vi "SpeedControlMotor4.vi"() -> ()   [LabVIEW 2014]
doc: "This example demonstrates how to simulate a general PID controller with a plant with noise."
uses:
  MyRIO Software/MyTypeDefs/EncoderController.ctl
  <vilib>/Analysis/3filter.llb/Filter Passband Type.ctl
  <vilib>/addons/control/pid/pid.llb/PID Percentage to EGU (DBL).vi
  <vilib>/addons/control/pid/pid.llb/PID Control Input Filter (DBL).vi
  <vilib>/addons/control/pid/pid.llb/PID (DBL).vi
  <vilib>/addons/control/pid/pid.llb/PID Output Rate Limiter (DBL).vi
  <vilib>/addons/control/pid/NI_PID_pid.lvlib
  <vilib>/ptbypt/NI_PtbyPt.lvlib
  <vilib>/Analysis/NI_AALBase.lvlib
panel:
  in  "Encoder 4 Controller":T1={"Sample time (uS)"=100000, "Reset"=FALSE}
  out "Sampling frequency (Hz)":dbl=4.0
  in  "cut-off frequency":dbl=6.0
  in  "order":i32=5
  in  "Filtering option":T2(ring)
  out "Manipulated variable (MV)":dbl(graph)=44.75756470842677
  in  "Output Limiter":bool
  in  "Output Rate (EGU/min)":dbl=10000.0 format="%#.2f"
  out "Unfiltered Speed(RPM)":dbl=55.83860880961906 format="%.4f"
  in  "Setpoint (RPM)":dbl(slide)=55.55555555555556 min=0.0 max=0.0 scale=-100.0..100.0
  out "MV:":dbl(slide)=38.025391430574594 scale=-100.0..100.0
  out "Speed (RPM):":dbl(slide)=55.83860880961906 scale=-100.0..100.0
  in  "PID gains":T3={"proportional gain (Kc)"=0.6, "integral time (Ti, min)"=0.01, "derivative time (Td, min)"=0.0} {"derivative time (Td, min)" format="%.3f"; "integral time (Ti, min)" format="%.3f"; "proportional gain (Kc)" format="%.3f"}
  in  "Controller Sampling Time":dbl=0.25 min=0.001 step=0.01 format="%#.3p"
  in  "Stop":bool
  out "System Monitor":T4(graph)={"Speed (RPM):"=55.13720442402905, "Setpoint (RPM)"=55.55555555555556, "Velocity RPM"=55.83860880961906}
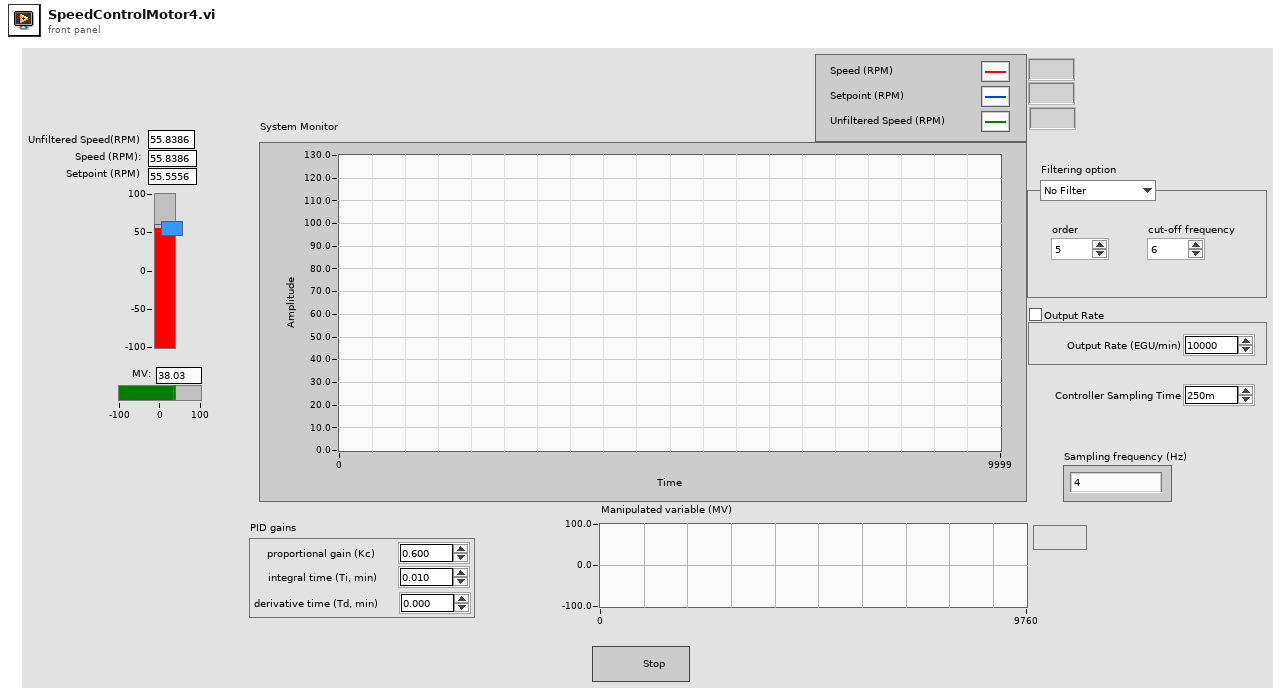
[diagram p1: front panel]
types:
  T1 = typedef "EncoderController.ctl" = cluster{"Sample time (uS)":u32, "Reset":bool}
  T2 = enum16{"No Filter", "PID FIR Filter", "Butterworth", "Chebyshev", "FIR Windowing", "Median"}
  T3 = cluster{"proportional gain (Kc)":dbl, "integral time (Ti, min)":dbl, "derivative time (Td, min)":dbl}
  T4 = cluster{"Speed (RPM):":dbl, "Setpoint (RPM)":dbl, "Velocity RPM":dbl}
  T5 = typedef "NI_AALBase.lvlib/Filter Passband Type.ctl" = enum32{"Lowpass", "Highpass", "Bandpass", "Bandstop"}
  T6 = cluster{bool, "Tick Count(uSec)":u32, "Counter Value":i32, "x-y":i32}
  T7 = typedef "EncoderIndicator.ctl" = cluster{"Position":dbl, "Velocity RPM":dbl, "Velocity RPS":dbl}
  T8 = cluster{"Speed (RPM):":dbl, "Setpoint (RPM)":dbl, dbl}
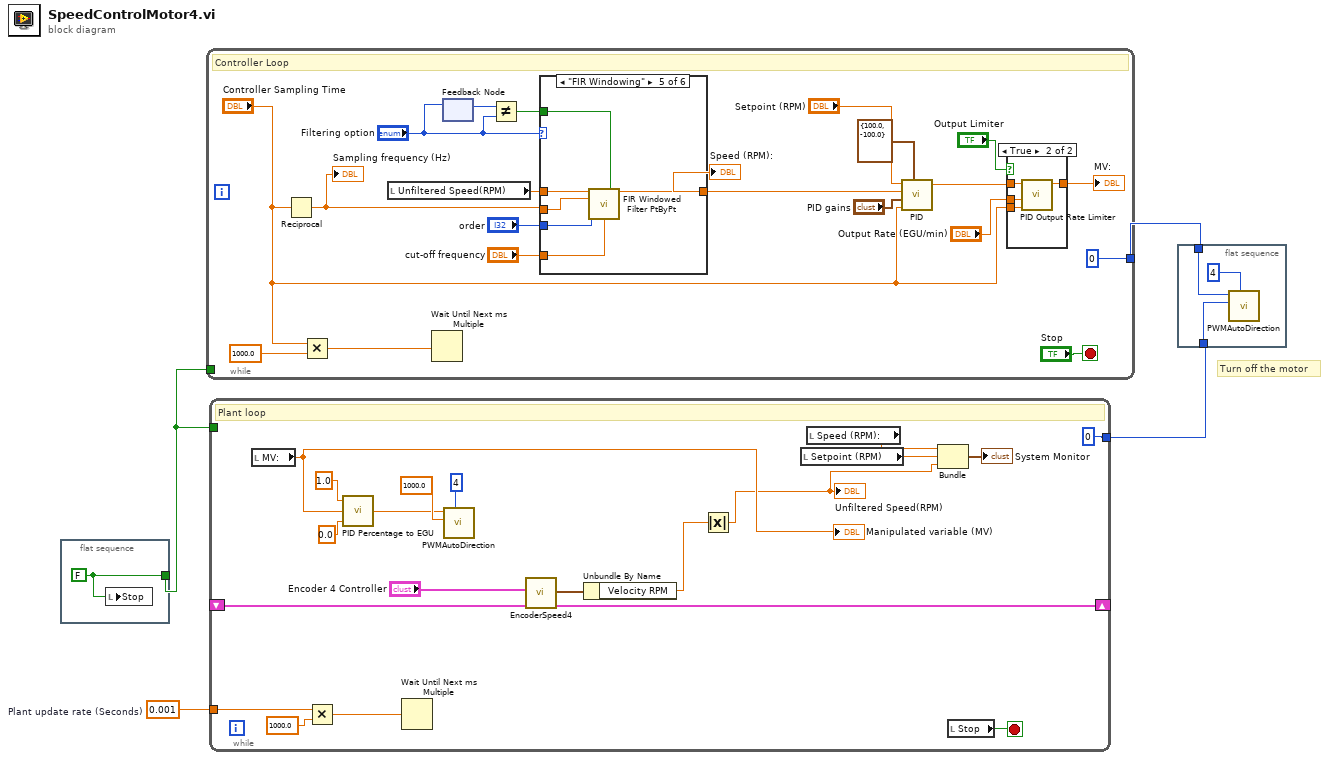
[diagram p0: block diagram]
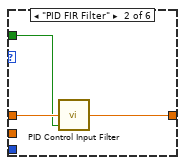
[diagram p3: hidden frame]
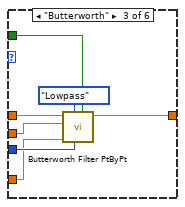
[diagram p4: hidden frame]
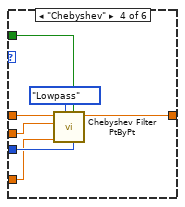
[diagram p5: hidden frame]
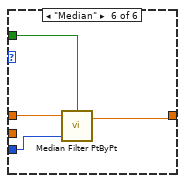
[diagram p6: hidden frame]
diagram:
  w4 = 0.001  # Plant update rate (Seconds)
  # "Turn off the motor"
  n1 = flat-sequence {
    tunnel: [w5] -> w3
    frame #0 {
      w5 = FALSE ("STOP")
      n2 = local write "Stop"(w5) -> ()
    }
  }
  n3 = while {
    tunnel: w3 -> [_]
    tunnel: [0] -> w2
    stop <- "Stop" stop-if-true
    # "Controller Loop"
    n4 = Reciprocal(x="Controller Sampling Time") -> (1/x=w24:dbl)
    "Sampling frequency (Hz)" <- w24
    n5 = Multiply(x="Controller Sampling Time", y=1000.0) -> (x*y=w25:dbl)
    n6 = local read "Unfiltered Speed(RPM)"() -> (w20:dbl)
    n7 = Wait Until Next ms Multiple(millisecond multiple=w25) -> ()  [unwired: 1 out]
    n8 = feedback-in #1("Filtering option") -> ()
    n9 = feedback #1() -> (w14:T2)  [unwired: 1 in]
    n10 = Not Equal?(x=w14, y="Filtering option") -> (x != y?=w12:bool)
    n11 = case shown="\"FIR Windowing\"" "Filtering option" {
      tunnel: [w26 w29 w36 w43 w49 w53] -> w21
      tunnel: w20 -> [w26 w28 w35 w42 w48 w52]
      tunnel: w24 -> [_ _ w34 w41 w47 _]
      tunnel: "order" -> [_ _ w32 w39 w46 w51]
      tunnel: "cut-off frequency" -> [_ _ w31 w38 w45 _]
      tunnel: w12 -> [_ w27 w30 w37 w44 w50]
      frame "No Filter", Default {
      }
      frame "PID FIR Filter" {
        n12 = call-poly <vilib>:"PID Control Input Filter.vi"("reinitialize? (F)"=w27, "input"=w28) -> ("output"=w29:dbl)  [unwired: 3 in]
      }
      frame "Butterworth" {
        n13 = call <vilib>:"Butterworth Filter PtByPt.vi"("initialize"=w30, "order"=w32, "filter type"=Filter_Passband_Type."Lowpass", "low cutoff freq: fl"=w31, "sampling freq: fs"=w34, "x"=w35) -> ("Filtered x"=w36:dbl)  [unwired: 3 in, 1 out]
      }
      frame "Chebyshev" {
        n14 = call <vilib>:"Chebyshev Filter PtByPt.vi"("order"=w39, "initialize"=w37, "filter type"=Filter_Passband_Type."Lowpass", "low cutoff freq: fl"=w38, "sampling freq: fs"=w41, "x"=w42) -> ("Filtered x"=w43:dbl)  [unwired: 4 in, 1 out]
      }
      frame "FIR Windowing" {
        n15 = call <vilib>:"FIR Windowed Filter PtByPt.vi"("x"=w48, "initialize"=w44, "sampling freq: fs"=w47, "taps"=w46, "low cutoff freq: fl"=w45) -> ("Filtered x"=w49:dbl)  [unwired: 9 in, 1 out]
      }
      frame "Median" {
        n16 = call <vilib>:"Median Filter PtByPt.vi"("initialize"=w50, "rank"=w51, "x"=w52) -> ("Filtered x"=w53:dbl)  [unwired: 1 in, 1 out]
      }
    }
    "Speed (RPM):" <- w21
    n17 = call-poly <vilib>:"PID.vi"("output range"=cluster{"output high":dbl, "output low":dbl} {"output high"=100.0, "output low"=-100.0}, "dt (s)"="Controller Sampling Time", "PID gains"="PID gains", "process variable"=w21, "setpoint"="Setpoint (RPM)") -> ("output"=w7:dbl)  [unwired: 5 in, 1 out]
    n18 = case shown="True" "Output Limiter" {
      tunnel: w7 -> [w54 w58]
      tunnel: "Controller Sampling Time" -> [_ w57]
      tunnel: [w54 w56] -> w6
      tunnel: "Output Rate (EGU/min)" -> [_ w55]
      frame False {
      }
      frame True {
        n19 = call-poly <vilib>:"PID Output Rate Limiter.vi"("dt (s)"=w57, "output rate (EGU/min)"=w55, "input (controller output)"=w58) -> ("output"=w56:dbl)  [unwired: 5 in, 1 out]
      }
    }
    "MV:" <- w6
  }
  n20 = while {
    tunnel: w4 -> [w72]
    tunnel: w3 -> [_]
    shift-right: [w71] -> _
    shift-left: _ -> [w70]
    tunnel: [0] -> w1
    stop <- w74 stop-if-true
    # "Plant loop"
    n21 = local read "MV:"() -> (w65:dbl)
    "Manipulated variable (MV)" <- w65
    n22 = Multiply(x=w72, y=1000.0) -> (x*y=w73:dbl)
    n23 = call-poly <vilib>:"PID Percentage to EGU.vi"("minimum (EGU)"=0.0, "% span"=w65, "maximum (EGU)"=1.0) -> ("output (EGU)"=w63:dbl)  [unwired: 1 in]
    n24 = Wait Until Next ms Multiple(millisecond multiple=w73) -> ()  [unwired: 1 out]
    n25 = call "PWMAutoDirection.vi"("Motor Select"=i8 4, "PWM Frequency"=1000.0, "DutyCycle"=w63) -> ()  [unwired: 8 in, 1 out]
    n26 = call "EncoderSpeed4.vi"("Cluster in"=w70, "Encoder 4 Controller"="Encoder 4 Controller") -> ("Cluster out"=w71:T6, "Encoder 4 Indicator"=w68:T7)  [unwired: 7 in, 1 out]
    n27 = Unbundle By Name(w68) -> ("Velocity RPM"=w60:dbl)
    n28 = Absolute Value(x=w60) -> (abs(x)=w59:dbl)
    "Unfiltered Speed(RPM)" <- w59
    n29 = local read "Setpoint (RPM)"() -> (w77:dbl)
    n30 = local read "Speed (RPM):"() -> (w75:dbl)
    n31 = Bundle("Speed (RPM):"=w75, "Setpoint (RPM)"=w77, w59) -> (→"System Monitor":T8)  [unwired: 1 in]
    n32 = local read "Stop"() -> (w74:bool)
  }
  n33 = flat-sequence {
    tunnel: w2 -> [w80]
    tunnel: w1 -> [w79]
    frame #0 {
      n34 = call "PWMAutoDirection.vi"("Motor Select"=i8 4, "PWM Frequency"=w79, "DutyCycle"=w80) -> ()  [unwired: 8 in, 1 out]
    }
  }
